vi "FP RT main.vi"() -> ()   [LabVIEW 2014]
uses:
  <vilib>/userdefined/High Color/IMAQdx.ctl
  <vilib>/myRIO/Instrument Drivers/Onboard IO/PWM/typedefs/PWM Reference.ctl
  <vilib>/myRIO/Common/Instrument Driver Framework/Utilities/typedefs/myRIO Generic Hardware Reference.ctl
  <vilib>/myRIO/Common/Instrument Driver Framework/Utilities/typedefs/Hardware Version Enum.ctl
  <vilib>/myRIO/Common/Instrument Driver Framework/Utilities/typedefs/myRIO v1.0 Reference.ctl
  <vilib>/myRIO/Common/Instrument Driver Framework/Utilities/typedefs/Generic FPGA Reference.ctl
  <vilib>/myRIO/Common/Instrument Driver Framework/myRIO v1.0/PWM/typedefs/PWM Channels Enum.ctl
  <vilib>/myRIO/Instrument Drivers/Onboard IO/PWM/typedefs/PWM Configuration.ctl
  <vilib>/userdefined/High Color/nirio_resource_hc.ctl
  <vilib>/myRIO/Instrument Drivers/Onboard IO/DIO/typedefs/DIO Reference.ctl
  <vilib>/myRIO/Common/Instrument Driver Framework/myRIO v1.0/DIO/typedefs/DIO Channels List.ctl
  <vilib>/myRIO/Common/Instrument Driver Framework/myRIO v1.0/DIO/typedefs/DIO Channels Enum.ctl
  <vilib>/myRIO/Instrument Drivers/Onboard IO/AI/typedefs/AI Reference.ctl
  <vilib>/myRIO/Common/Instrument Driver Framework/myRIO v1.0/AI/typedefs/AI Channels List.ctl
  <vilib>/myRIO/Common/Instrument Driver Framework/myRIO v1.0/AI/typedefs/AI Channels Enum.ctl
  <vilib>/myRIO/Common/Instrument Driver Framework/Utilities/typedefs/Analog Scaling Constants List.ctl
  <vilib>/myRIO/Common/Instrument Driver Framework/Utilities/typedefs/Analog Scaling Constants.ctl
  <vilib>/myRIO/Common/Instrument Driver Framework/myRIO v1.0/PWM/vis/myRIO v1.1 Open PWM.vi
  <vilib>/myRIO/Common/Instrument Driver Framework/myRIO v1.0/DIO/vis/myRIO v1.1 Open DIO.vi
  <vilib>/myRIO/Common/Instrument Driver Framework/myRIO v1.0/AI/vis/myRIO v1.1 Open AI.vi
  <vilib>/myRIO/Common/Instrument Driver Framework/Utilities/vis/Validate Channels.vi
  <vilib>/myRIO/Common/Instrument Driver Framework/myRIO v1.0/PWM/vis/myRIO v1.0 Reserve PWM.vi
  <vilib>/myRIO/Common/Instrument Driver Framework/myRIO v1.0/DIO/vis/myRIO v1.0 Reserve DIO.vi
  <vilib>/myRIO/Common/Instrument Driver Framework/myRIO v1.0/AI/vis/myRIO v1.0 Reserve AI.vi
  <vilib>/myRIO/Common/Instrument Driver Framework/myRIO v1.0/PWM/vis/myRIO v1.0 Close PWM.vi
  <vilib>/myRIO/Common/Instrument Driver Framework/myRIO v1.0/DIO/vis/myRIO v1.0 Close DIO.vi
  <vilib>/myRIO/Common/Instrument Driver Framework/myRIO v1.0/AI/vis/myRIO v1.0 Close AI.vi
  <vilib>/myRIO/Common/Instrument Driver Framework/myRIO v1.0/PWM/vis/myRIO v1.0 Build MUX Configuration PWM.vi
  <vilib>/myRIO/Common/Instrument Driver Framework/myRIO v1.0/Resource Manager/vis/myRIO v1.0 Reserve Channel List.vi
  <vilib>/myRIO/Common/Instrument Driver Framework/myRIO v1.0/DIO/vis/myRIO v1.0 Build MUX Configuration DIO.vi
  <vilib>/myRIO/Common/Instrument Driver Framework/myRIO v1.0/AI/vis/myRIO v1.0 Build MUX Configuration AI.vi
  <vilib>/myRIO/Common/Instrument Driver Framework/myRIO v1.0/PWM/vis/myRIO v1.0 Unreserve PWM.vi
  <vilib>/myRIO/Common/Instrument Driver Framework/myRIO v1.0/DIO/vis/myRIO v1.0 Unreserve DIO.vi
  <vilib>/myRIO/Common/Instrument Driver Framework/myRIO v1.0/AI/vis/myRIO v1.0 Unreserve AI.vi
  <vilib>/myRIO/Common/Instrument Driver Framework/myRIO v1.0/Resource Manager/vis/myRIO v1.0 Create Configuration List.vi
  <vilib>/myRIO/Common/Instrument Driver Framework/myRIO v1.0/Resource Manager/vis/myRIO v1.0 Reserve Channel.vi
  <vilib>/myRIO/Common/Instrument Driver Framework/myRIO v1.0/Resource Manager/vis/myRIO v1.0 Unreserve Channel.vi
  <vilib>/myRIO/Common/Instrument Driver Framework/myRIO v1.0/Resource Manager/vis/myRIO v1.0 Unreserve Channel List.vi
  <vilib>/myRIO/Common/Instrument Driver Framework/myRIO v1.0/Resource Manager/vis/myRIO v1.0 Build Mutex Name.vi
  <vilib>/Utility/VariantDataType/GetNumericInfo.vi
  <vilib>/Utility/error.llb/Error Cluster From Error Code.vi
  <vilib>/myRIO/Common/Instrument Driver Framework/myRIO v1.0/myRIO v1.1 Open.vi
  <vilib>/myRIO/Common/Instrument Driver Framework/myRIO v1.0/AI/vis/myRIO v1.0 Get Scaling Constants AI.vi
  <vilib>/myRIO/Common/Instrument Driver Framework/Utilities/vis/IO Manager.vi
  <vilib>/myRIO/Common/Instrument Driver Framework/Utilities/vis/Configuration Manager.vi
  <vilib>/myRIO/Common/Instrument Driver Framework/myRIO v1.0/myRIO v1.0 Close.vi
  <vilib>/myRIO/Common/Instrument Driver Framework/myRIO v1.0/Resource Manager/vis/myRIO v1.0 Configure IO.vi
  <vilib>/myRIO/Common/Instrument Driver Framework/myRIO v1.0/AI/vis/myRIO v1.0 Read AI.vi
  <vilib>/myRIO/Common/Instrument Driver Framework/myRIO v1.0/DIO/vis/myRIO v1.0 Write DIO.vi
  <vilib>/myRIO/Common/Instrument Driver Framework/myRIO v1.0/PWM/vis/myRIO v1.0 Write PWM.vi
  <vilib>/myRIO/Common/Instrument Driver Framework/myRIO v1.0/PWM/vis/myRIO v1.0 Shutdown PWM.vi
  <vilib>/myRIO/Common/Instrument Driver Framework/myRIO v1.0/DIO/vis/myRIO v1.0 Shutdown DIO.vi
  <vilib>/myRIO/Instrument Drivers/Onboard IO/AI/vis/myRIO AI Open.xnode
  <vilib>/myRIO/Instrument Drivers/Onboard IO/DIO/vis/myRIO DIO Open.xnode
  <vilib>/myRIO/Instrument Drivers/Onboard IO/PWM/vis/myRIO PWM Open.xnode
  <vilib>/vision/driver/NI_Vision_Acquisition_Software.lvlib
  <vilib>/myRIO/Instrument Drivers/Onboard IO/AI/AI.lvlib
  <vilib>/myRIO/Instrument Drivers/Onboard IO/DIO/DIO.lvlib
  <vilib>/myRIO/Instrument Drivers/Onboard IO/PWM/PWM.lvlib
panel:
  in  "Tab Control":T1(tab)
  out "GLED":bool
  out "BLED":bool
  out "RLED":bool
  out "BW Image":T2(plugin-control)
  in  "stop":bool
  out "Midbrain?":bool
  out "Rudder":dbl(knob) min=-45.0 max=45.0 step=1.0 scale=-45.0..45.0
  out "Speed":dbl(knob) min=-9.0 max=9.0 step=1.0 scale=-50.0..50.0
  out "Hindbrain?":bool
  out "Forebrain?":bool
  out "Battery Dead?":bool
  out "Complete?":bool=TRUE
  out "Arbiter Graph":cluster{dbl, dbl, dbl[]}(graph)
  in  "Session In":T3="cam0"
  out "Color Image":T2(plugin-control)
  out "Nb Circles":i32
  out "UDP Time Out?":bool
  in  "Tug letter":string="T"
  in  "Run?":bool
  in  "MSpeed":dbl(slide) scale=-50.0..50.0 scale format="%#.1g"
  in  "MHeading":dbl(slide) scale=-45.0..45.0 scale format="%_1f"
  in  "Manual?":bool
  out "Camera Data":T4(array[cluster])
  out "Boat Status":T5={"GPS"={"X pos"=0, "Y pos"=0, "Heading"=0.0}, "IR Sensors"=[{"Name"="Bow", "Angle"=0.0, "Distance"=0.0}], "MOT BAT"=7.2, "RIO BAT"=7.2}
  out "GPS?":bool
  out "Act Com":T6
  out "Forebrain ACT":dbl[](array[numeric])
  out "IR Sensors":T7(array[cluster])
  out "GPS":cluster{"X pos":i32, "Y pos":i32, "Heading":dbl}
  out "RED LED":bool
  out "GREEN LED":bool
  out "BLUE LED":bool
  in  "MDF":T8(array[cluster])=[{"Type"=enum."Start", "X"=250, "Y"=250, "Speed"=0, "Behaviors"=enum."Open Water Transit"}, {"Type"=enum."Waypoint", "X"=400, "Y"=100, "Speed"=20, "Behaviors"=enum."P-Wall Follow"}, {"Type"=enum."Waypoint", "X"=250, "Y"=250, "Speed"=20, "Behaviors"=enum."Open Water Transit"}, {"Type"=enum."Waypoint", "X"=250, "Y"=400, "Speed"=20, "Behaviors"=enum."Open Water Transit"}, {"Type"=enum."Waypoint", "X"=100, "Y"=400, "Speed"=20, "Behaviors"=enum."Open Water Transit"}, {"Type"=enum."End", "X"=250, "Y"=250, "Speed"=0, "Behaviors"=enum."Open Water Transit"}]
  out "GPS Initial":cluster{"X pos":i32, "Y pos":i32, "Heading":dbl}
  in  "Old Y Position":i32
  in  "Old X Position":i32
  out "Invalid Pos?":bool
  out "error out":errorcluster
  out "Forebrain Comd":T9
  out "Debug IR \nRaw \nReadings":T7(array[cluster])
  out "Boat Speed":dbl format="%#_15g"
  out "size(s)":i32
  out "MDF Active":T8(array[cluster])
  out "MDF INDEX":i32
  # "To start the Tug, press the \">\" key in the tool bar.\n\nPress the Run? control to start the Mission.\n\nWhen complete the Complete? indicator will light.\n\nIf the Run? is not pressed again, the mission will start again.\n\nAlways press the STOP button to end the operation!!!!!!!!!!!!!"
  # "Press the Manual? button to control\nthe Tug from the sliders"
  # "Stuck indicates that\nthe boat is not moving."
  # "Enter the Letter\nof  your Tug"
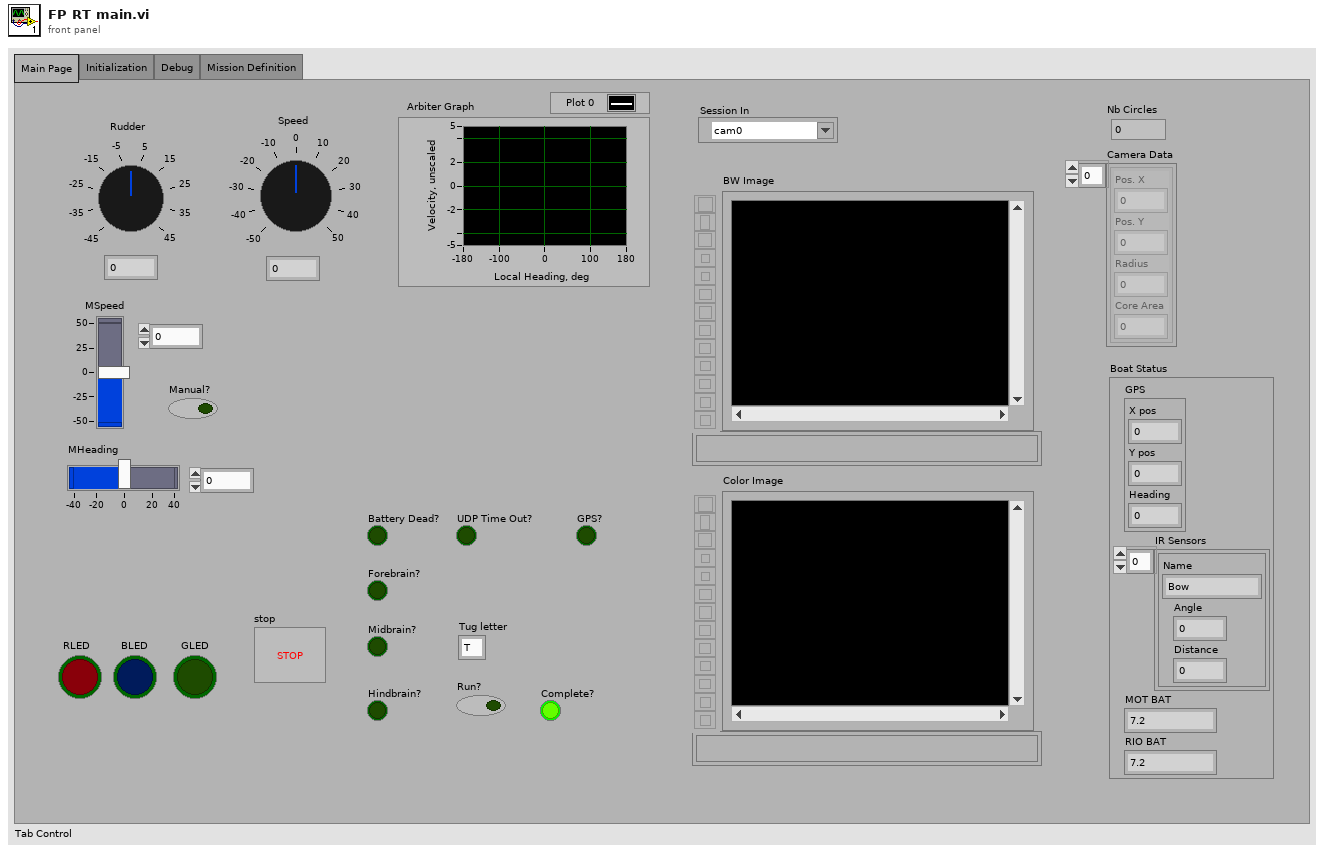
[diagram p1: front panel]
types:
  T1 = enum32{"Main Page", "Initialization", "Debug", "Mission Definition"}
  T2 = typedef "IMAQ Image.ctl" = refnum<image>
  T3 = typedef "IMAQdx.ctl" = refnum<k21>
  T4 = cluster{"Pos. X":i32, "Pos. Y":i32, "Radius":i32, "Core Area":i32}[]
  T5 = cluster{"GPS":cluster{"X pos":i32, "Y pos":i32, "Heading":dbl}, "IR Sensors":cluster{"Name":string, "Angle":dbl, "Distance":dbl}[], "MOT BAT":dbl, "RIO BAT":dbl}
  T6 = cluster{"Desired Local\nHeading":dbl, "Desired\nSpeed":dbl}
  T7 = cluster{"Name":string, "Angle":dbl, "Distance":dbl}[]
  T8 = cluster{"Type":enum16{"Start", "Waypoint", "End"}, "X":i32, "Y":i32, "Speed":i32, "Behaviors":enum16{"Open Water Transit", "P-Wall Follow", "S-Wall Follow", "Dock"}}[]
  T9 = cluster{"Behaviors":enum16{"Open Water Transit", "P-Wall Follow", "S-Wall Follow", "Dock"}, "Behavior\nVelocity":dbl}
  T10 = typedef "nirio_resource_hc.ctl" = tag
  T11 = typedef "Hardware Version Enum.ctl" = enum16{"Unknown", "myRIO-1900", "myRIO-1950"}
  T12 = typedef "Image Type" = u32
  T13 = enum16{"Open Water Transit", "P-Wall Follow", "S-Wall Follow", "Dock"}
  T14 = typedef "PWM.lvlib/PWM Reference.ctl" = cluster{"myRIO Reference":T15, "PWM Channels Enum":T18, "PWM Configuration":T19}
  T15 = typedef "myRIO Generic Hardware Reference.ctl" = cluster{"myRIO Model":T11, "myRIO Hardware Reference":T16}
  T16 = typedef "myRIO v1.0 Reference.ctl" = cluster{"Generic FPGA Reference":T17, "Allow multiple opens":bool}
  T17 = typedef "Generic FPGA Reference.ctl" = refnum<k20>
  T18 = typedef "PWM Channels Enum.ctl" = enum16{"Not Connected", "C/PWM0", "C/PWM1", "A/PWM0", "A/PWM1", "A/PWM2", "B/PWM0", "B/PWM1", "B/PWM2"}
  T19 = typedef "PWM.lvlib/PWM Configuration.ctl" = cluster{"Frequency":dbl, "Duty Cycle":dbl}
  T20 = typedef "DIO.lvlib/DIO Reference.ctl" = cluster{"myRIO Reference":T15, "DIO Channels List":T21}
  T21 = typedef "DIO Channels List.ctl" = T22[]
  T22 = typedef "DIO Channels Enum.ctl" = enum16{"Not Connected", "C/DIO0", "C/DIO1", "C/DIO2", "C/DIO3", "C/DIO4", "C/DIO5", "C/DIO6", "C/DIO7", "A/DIO0", "A/DIO1", "A/DIO2", "A/DIO3", "A/DIO4", "A/DIO5", "A/DIO6", "A/DIO7", "A/DIO8", "A/DIO9", "A/DIO10", "A/DIO11", "A/DIO12", "A/DIO13", "A/DIO14", "A/DIO15", "B/DIO0", "B/DIO1", "B/DIO2", "B/DIO3", "B/DIO4", "B/DIO5", "B/DIO6", "B/DIO7", "B/DIO8", "B/DIO9", "B/DIO10", "B/DIO11", "B/DIO12", "B/DIO13", "B/DIO14", "B/DIO15", "LED0", "LED1", "LED2", "LED3", "Button0"}
  T23 = typedef "AI.lvlib/AI Reference.ctl" = cluster{"myRIO Reference":T15, "AI Channels List":T24, "AI Scaling Constants List":T26}
  T24 = typedef "AI Channels List.ctl" = T25[]
  T25 = typedef "AI Channels Enum.ctl" = enum16{"Not Connected", "AudioIn/Left", "AudioIn/Right", "C/AI0", "C/AI1", "A/AI0", "A/AI1", "A/AI2", "A/AI3", "B/AI0", "B/AI1", "B/AI2", "B/AI3"}
  T26 = typedef "Analog Scaling Constants List.ctl" = T27[]
  T27 = typedef "Analog Scaling Constants.ctl" = cluster{"LSB Weight (Volts)":dbl, "Offset (Volts)":dbl, "Signed?":bool}
  T28 = cluster{"Obs Avoid Array":dbl[], "P-Wall Array":dbl[], "S-Wall Array":dbl[], "Unstuck Array":dbl[]}
  T29 = cluster{"regular expression":string, i32, i32, i32}
  T30 = cluster{"Behaviors":enum16{"Open Water Transit", "P-Wall Follow", "S-Wall Follow", "Dock"}, dbl}
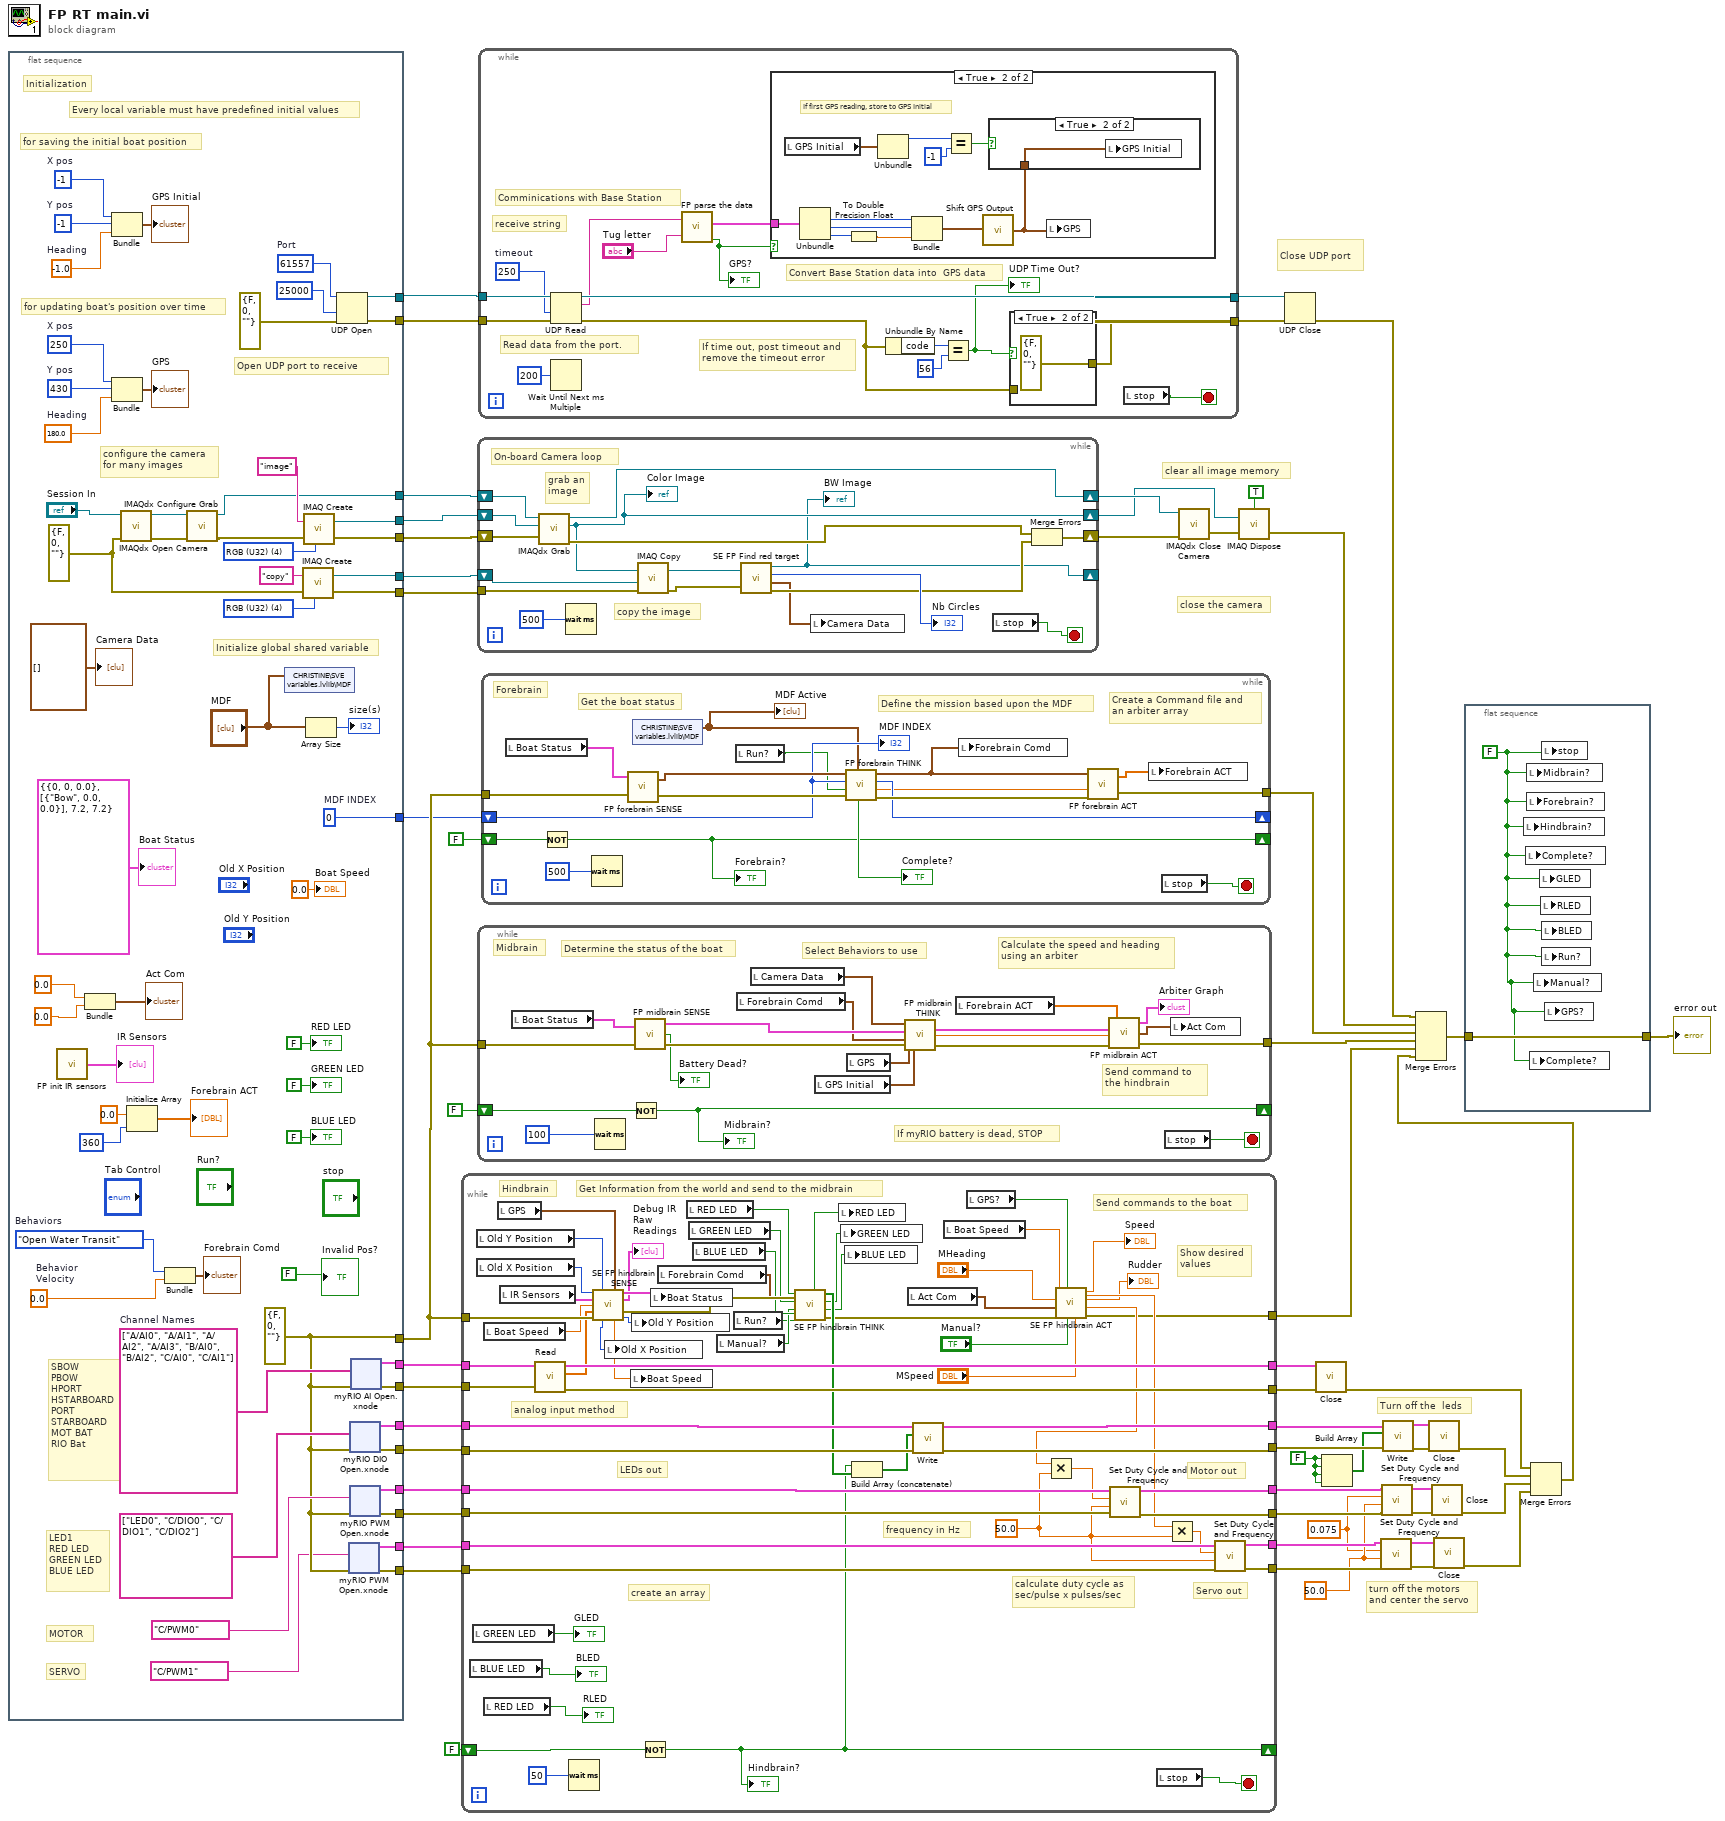
[diagram p0: block diagram]
diagram:
  w5 = 0.075
  w4 = FALSE
  w6 = 50.0
  # "Turn off the  leds"
  # "turn off the motors\nand center the servo"
  # "Close UDP port"
  # "clear all image memory"
  # "close the camera"
  n1 = flat-sequence {
    tunnel: [w74] -> w54
    tunnel: [w109] -> w51
    tunnel: [w100] -> w50
    tunnel: [w99] -> w49
    tunnel: [w98] -> w48
    tunnel: [w94] -> w41
    tunnel: [w93] -> w42
    tunnel: [w89] -> w36
    tunnel: [w88] -> w37
    tunnel: [w82] -> w34
    tunnel: [w81] -> w33
    tunnel: [w79] -> w29
    tunnel: [w78] -> w30
    tunnel: [w76] -> w28
    tunnel: [w75] -> w27
    tunnel: [w72] -> w26
    tunnel: [w71] -> w25
    frame #0 {
      w59 = -1  # Y pos
      w60 = -1  # X pos
      w61 = -1.0  # Heading
      w83 = tag[] ["A/AI0", "A/AI1", "A/AI2", "A/AI3", "B/AI0", "B/AI2", "C/AI0", "C/AI1"]  # Channel Names
      w85 = 430  # Y pos
      w86 = 250  # X pos
      w87 = 180.0  # Heading
      w92 = u16 61557  # Port
      w97 = T12 4 items=["Grayscale (U8)", "Grayscale (I16)", "Grayscale (SGL)", "Complex (CSG)", "RGB (U32)", "HSL (U32)", "RGB (U64)", "Grayscale (U16)"] ("Image Type")
      w95 = errorcluster {"status"=FALSE, "code"=0, "source"=""} ("error in")
      w105 = T12 4 items=["Grayscale (U8)", "Grayscale (I16)", "Grayscale (SGL)", "Complex (CSG)", "RGB (U32)", "HSL (U32)", "RGB (U64)", "Grayscale (U16)"] ("Image Type")
      w74 = errorcluster {"status"=FALSE, "code"=0, "source"=""} ("error out")
      w109 = 0  # MDF INDEX
      w113 = 0.0  # Behavior Velocity
      w108 = T13."Open Water Transit"  # Behaviors
      # "for saving the initial boat position"
      # "Initialize global shared variable"
      # "LED1\nRED LED\nGREEN LED\nBLUE LED"
      # "SERVO"
      # "MOTOR"
      # "SBOW\nPBOW\nHPORT\nHSTARBOARD\nPORT\nSTARBOARD\nMOT BAT\nRIO Bat"
      # "for updating boat's position over time"
      # "Open UDP port to receive"
      # "configure the camera\nfor many images"
      # "Every local variable must have predefined initial values"
      # "Initialization"
      n2 = call "FP init IR sensors.vi"() -> ("IR Sensors"=→"IR Sensors":T7)  [unwired: 1 in]
      n3 = Bundle(0.0, 0.0) -> (→"Act Com":cluster{dbl, dbl})  [unwired: 1 in]
      n4 = Bundle("X pos"=w60, "Y pos"=w59, "Heading"=w61) -> (→"GPS Initial":cluster{"X pos":i32, "Y pos":i32, "Heading":dbl})  [unwired: 1 in]
      n5 = Bundle("X pos"=w86, "Y pos"=w85, "Heading"=w87) -> (→"GPS":cluster{"X pos":i32, "Y pos":i32, "Heading":dbl})  [unwired: 1 in]
      n6 = call <vilib>:"IMAQdx Open Camera.vi"("error in"=w95, "Session In"="Session In") -> ("error out"=w102:errorcluster, "Session Out"=w101:T3)  [unwired: 1 in, 7 out]
      n7 = Initialize Array(0.0 ("element"), 360 ("dimension size")) -> (→"Forebrain ACT":dbl[])
      n8 = Bundle("Behaviors"=w108, "Behavior\nVelocity"=w113) -> (→"Forebrain Comd":T9)  [unwired: 1 in]
      n9 = call <vilib>:"IMAQdx Configure Grab.vi"("error in"=w102, "Session In"=w101) -> ("error out"=w106:errorcluster, "Session Out"=w98:T3)  [unwired: 8 out]
      n10 = shared-variable "CHRISTINE\\SVE variables.lvlib\\MDF"("MDF") -> ()  [unwired: 1 in, 1 out]
      n11 = call "IMAQ Create"("Image Name"="copy", "Image Type"=w97, "error in (no error)"=w95) -> ("New Image"=w93:T2, "error out"=w94:errorcluster)  [unwired: 2 in]
      n12 = call "IMAQ Create"("Image Name"="image", "Image Type"=w105, "error in (no error)"=w106) -> ("New Image"=w99:T2, "error out"=w100:errorcluster)  [unwired: 1 in, 1 out]
      n13 = Array Size(array="MDF") -> (size(s)=→"size(s)":i32)
      n14 = UDP Open(8:errorcluster {"status"=FALSE, "code"=0, "source"=""} ("error in"), 9:25000 ("timeout ms (25000)"), 11:w92) -> (port=w89:refnum<k16>, 0:w88:errorcluster)  [unwired: 2 in, 1 out]
      n15 = xnode "myRIO PWM Open.xnode"("error in (no error)"=w74, "Channel Name"=tag "C/PWM1") -> ("error out"=w72:errorcluster, "PWM Ref Out"=w71:T14)  [unwired: 1 in]
      n16 = xnode "myRIO DIO Open.xnode"("error in (no error)"=w74, "Channel Names"=tag[] ["LED0", "C/DIO0", "C/DIO1", "C/DIO2"]) -> ("error out"=w79:errorcluster, "DIO Ref Out"=w78:T20)  [unwired: 1 in]
      n17 = xnode "myRIO PWM Open.xnode"("error in (no error)"=w74, "Channel Name"=tag "C/PWM0") -> ("error out"=w76:errorcluster, "PWM Ref Out"=w75:T14)  [unwired: 1 in]
      n18 = xnode "myRIO AI Open.xnode"("error in (no error)"=w74, "Channel Names"=w83) -> ("error out"=w82:errorcluster, "AI Ref Out"=w81:T23)  [unwired: 1 in]
      "Invalid Pos?" <- FALSE
      "RED LED" <- FALSE ("RED LED")
      "GREEN LED" <- FALSE ("GREEN LED")
      "BLUE LED" <- FALSE ("WHITE LED")
      "Camera Data" <- T4 [] ("Camera Data")
      "Boat Status" <- T5 {"GPS"={"X pos"=0, "Y pos"=0, "Heading"=0.0}, "IR Sensors"=[{"Name"="Bow", "Angle"=0.0, "Distance"=0.0}], "MOT BAT"=7.2, "RIO BAT"=7.2} ("Boat Status 2")
      "Boat Speed" <- 0.0 ("Boat Speed")
    }
  }
  n19 = while {
    tunnel: w54 -> [w243]
    shift-right: [w207] -> _
    shift-left: FALSE -> [w232]
    tunnel: w34 -> [w240]
    tunnel: w33 -> [w239]
    tunnel: [w238] -> w32
    tunnel: [w237] -> w31
    tunnel: w30 -> [w235]
    tunnel: w29 -> [w236]
    tunnel: [w234] -> w11
    tunnel: [w233] -> w8
    tunnel: w28 -> [w230]
    tunnel: w27 -> [w231]
    tunnel: [w229] -> w20
    tunnel: [w228] -> w17
    tunnel: w26 -> [w227]
    tunnel: [w226] -> w24
    tunnel: w25 -> [w225]
    tunnel: [w224] -> w22
    tunnel: [w186] -> w1
    stop <- w245 stop-if-true
    w219 = 50.0
    # "create an array"
    # "frequency in Hz"
    # "calculate duty cycle as\nsec/pulse x pulses/sec"
    # "Show desired\nvalues"
    # "Motor out"
    # "Servo out"
    # "LEDs out"
    # "analog input method"
    # "Send commands to the boat"
    # "Get Information from the world and send to the midbrain"
    # "Hindbrain"
    n20 = local read "BLUE LED"() -> (→"BLED":bool)
    n21 = local read "GREEN LED"() -> (→"GLED":bool)
    n22 = local read "Old Y Position"() -> (w191:i32)
    n23 = local read "Old X Position"() -> (w192:i32)
    n24 = local read "Boat Speed"() -> (w188:dbl)
    n25 = local read "RED LED"() -> (→"RLED":bool)
    n26 = local read "GPS"() -> (w241:cluster{"X pos":i32, "Y pos":i32, "Heading":dbl})
    n27 = local read "IR Sensors"() -> (w205:T7)
    n28 = call <vilib>:"Read.vi"("error in (no error)"=w240, "AI Ref In"=w239) -> ("error out"=w238:errorcluster, "Values"=w223:dbl[], "AI Ref Out"=w237:T23)  [unwired: 7 in]
    n29 = Wait (ms)(milliseconds to wait=u32 50) -> ()  [unwired: 1 out]
    n30 = call "SE FP hindbrain SENSE.vi"("Old X Position"=w192, "Old Y Position"=w191, "GPS"=w241, "IR Sensors"=w205, "Old Speed of Boat\nin Pixels/Sec"=w188, "Analog Input Values"=w223, "error in"=w243) -> ("Boat Status"=w206:T5, "IR Sensors 2"=→"Debug IR \nRaw \nReadings":T7, "error out"=w242:errorcluster, "New X Position"=w190:i32, "New Speed of Boat\nin Pixels/Sec"=w194:dbl, "New Y Position"=w189:i32)  [unwired: 3 in]
    n31 = local write "Old X Position"(w190) -> ()
    n32 = local write "Boat Speed"(w194) -> ()
    n33 = local write "Old Y Position"(w189) -> ()
    n34 = Not(x=w232) -> (.not. x?=w207:bool)
    "Hindbrain?" <- w207
    n35 = local write "Boat Status"(w206) -> ()
    n36 = local read "Forebrain Comd"() -> (w204:T9)
    n37 = local read "RED LED"() -> (w210:bool)
    n38 = local read "GREEN LED"() -> (w209:bool)
    n39 = local read "BLUE LED"() -> (w208:bool)
    n40 = local read "Manual?"() -> (w200:bool)
    n41 = local read "Run?"() -> (w195:bool)
    n42 = call "SE FP hindbrain THINK.vi"("error in"=w242, "BLUE LED"=w208, "Forebrain Comd"=w204, "RUN?"=w195, "MANUAL"=w200, "GREEN LED"=w209, "RED LED"=w210) -> ("error out"=w187:errorcluster, "BLUE LED OUT"=w201:bool, "GREEN LED OUT"=w202:bool, "LED array"=w212:bool[], "RED LED OUT"=w203:bool)
    n43 = local write "RED LED"(w203) -> ()
    n44 = local write "GREEN LED"(w202) -> ()
    n45 = local write "BLUE LED"(w201) -> ()
    n46 = Build Array (concatenate)(w207, w212) -> (w211:bool[])
    n47 = local read "Act Com"() -> (w216:T6)
    n48 = call <vilib>:"Write.vi"("error in (no error)"=w236, "Values"=w211, "DIO Ref In"=w235) -> ("error out"=w234:errorcluster, "DIO Ref Out"=w233:T20)  [unwired: 6 in]
    n49 = local read "Boat Speed"() -> (w193:dbl)
    n50 = local read "GPS?"() -> (w185:bool)
    n51 = call "SE FP hindbrain ACT.vi"("MSpeed"="MSpeed", "Manual?"="Manual?", "GPS?"=w185, "error in"=w187, "Act Com"=w216, "MHeading"="MHeading", "Current Boat Speed"=w193) -> ("error out"=w186:errorcluster, "Speed"=w222:dbl, "Desired \nRudder"=→"Rudder":dbl, "Desired\nSpeed"=→"Speed":dbl, "Rudder"=w220:dbl)
    n52 = Multiply(x=w222, y=w219) -> (x*y=w221:dbl)
    n53 = call <vilib>:"Set Duty Cycle and Frequency.vi"("error in (no error)"=w230, "Frequency [Hz]"=w219, "Duty Cycle"=w221, "PWM Ref In"=w231) -> ("error out"=w229:errorcluster, "PWM Ref Out"=w228:T14)  [unwired: 5 in]
    n54 = local read "stop"() -> (w245:bool)
    n55 = Multiply(x=w220, y=w219) -> (x*y=w218:dbl)
    n56 = call <vilib>:"Set Duty Cycle and Frequency.vi"("error in (no error)"=w227, "Frequency [Hz]"=w219, "Duty Cycle"=w218, "PWM Ref In"=w225) -> ("error out"=w226:errorcluster, "PWM Ref Out"=w224:T14)  [unwired: 5 in]
  }
  n57 = while {
    shift-right: [w249] -> w46
    shift-left: w50 -> [w261]
    shift-right: [w248] -> w44
    shift-left: w49 -> [w260]
    shift-right: [w253] -> w45
    shift-left: w48 -> [w259]
    tunnel: w41 -> [w257]
    shift-right: [w247] -> _
    shift-left: w42 -> [w256]
    stop <- w262 stop-if-true
    # "grab an\nimage"
    # "copy the image"
    # "On-board Camera loop"
    n58 = call <vilib>:"IMAQdx Grab.vi"("error in"=w261, "Image In"=w260, "Session In"=w259) -> ("error out"=w250:errorcluster, "Image Out"=w248:T2, "Session Out"=w253:T3)  [unwired: 5 in, 1 out]
    "Color Image" <- w248
    n59 = Wait (ms)(milliseconds to wait=u32 500) -> ()  [unwired: 1 out]
    n60 = call "IMAQ Copy"("error in (no error)"=w257, "Image Dst"=w256, "Image Src"=w248) -> ("error out"=w255:errorcluster, "Image Dst Out"=w254:T2)  [unwired: 3 in]
    n61 = call "SE FP Find red target.vi"("Image In"=w254, "error in (no error)"=w255) -> ("Image Dst Out"=w247:T2, "Nb Circles (Circle Detection 1)"=→"Nb Circles":i32, "Camera Data"=w246:T4, "error out"=w251:errorcluster)
    "BW Image" <- w247
    n62 = local write "Camera Data"(w246) -> ()
    n63 = local read "stop"() -> (w262:bool)
    n64 = Merge Errors(w250, w251) -> (w249:errorcluster)
  }
  n65 = while {
    shift-right: [w270] -> _
    shift-left: FALSE -> [w281]
    tunnel: w54 -> [w280]
    tunnel: [w274] -> w56
    stop <- w282 stop-if-true
    # "If myRIO battery is dead, STOP"
    # "Send command to \nthe hindbrain"
    # "Calculate the speed and heading\nusing an arbiter"
    # "Select Behaviors to use"
    # "Determine the status of the boat"
    # "Midbrain"
    n66 = local read "Boat Status"() -> (w265:T5)
    n67 = Wait (ms)(milliseconds to wait=u32 100) -> ()  [unwired: 1 out]
    n68 = Not(x=w281) -> (.not. x?=w270:bool)
    "Midbrain?" <- w270
    n69 = call "FP midbrain SENSE.vi"("Boat Status"=w265, "error in"=w280) -> ("IR Sensors"=w268:T7, "Battery\nDead?"=→"Battery Dead?":bool, "error out"=w278:errorcluster)
    n70 = local read "Forebrain Comd"() -> (w267:T9)
    n71 = local read "Camera Data"() -> (w266:T4)
    n72 = local read "GPS Initial"() -> (w264:cluster{"X pos":i32, "Y pos":i32, "Heading":dbl})
    n73 = local read "GPS"() -> (w263:cluster{"X pos":i32, "Y pos":i32, "Heading":dbl})
    n74 = call "FP midbrain THINK.vi"("Camera Data"=w266, "error in"=w278, "IR Sensors"=w268, "Forebrain Comd"=w267, "GPS  Initial"=w264, "GPS"=w263) -> ("Behavior arrays"=w275:T28, "Behavior\nVelocity OUT"=w272:dbl, "error out"=w277:errorcluster)
    n75 = local read "Forebrain ACT"() -> (w273:dbl[])
    n76 = call "FP midbrain ACT.vi"("error in"=w277, "Behavior\nVelocity"=w272, "Behavior arrays"=w275, "Forebrain ACT"=w273) -> ("error out"=w274:errorcluster, "Act Com"=w279:T6, "Waveform Graph"=→"Arbiter Graph":cluster{dbl, dbl, dbl[]})
    n77 = local read "stop"() -> (w282:bool)
    n78 = local write "Act Com"(w279) -> ()
  }
  n79 = while {
    tunnel: w37 -> [w297]
    tunnel: w36 -> [w296]
    tunnel: [w295] -> w39
    tunnel: [w290] -> w38
    stop <- w287 stop-if-true
    w289 = 250  # timeout
    # "Convert Base Station data into  GPS data"
    # "Comminications with Base Station"
    # "receive string"
    # "If time out, post timeout and\nremove the timeout error"
    # "Read data from the port."
    n80 = UDP Read(connection ID=w296, timeout ms (25000)=w289, 8:w297) -> (data out=w284:string, error out=w291:errorcluster, 3:w295:refnum<k16>)  [unwired: 1 in, 2 out]
    n81 = Wait Until Next ms Multiple(millisecond multiple=u32 200) -> ()  [unwired: 1 out]
    n82 = call "FP parse the data.vi"("Nav String"=w284, "Tug"="Tug letter") -> ("Tug Location"=w285:T29, "Valid?"=w283:bool)  [unwired: 2 out]
    "GPS?" <- w283
    n83 = case shown="True" w283 {
      tunnel: w285 -> [_ w308]
      frame False {
      }
      frame True {
        # "If first GPS reading, store to GPS Initial"
        n84 = local read "GPS Initial"() -> (w301:cluster{"X pos":i32, "Y pos":i32, "Heading":dbl})
        n85 = Unbundle(w308) -> (w307:i32, w306:i32, w304:i32)  [unwired: 1 out]
        n86 = To Double Precision Float(number=w304) -> (double precision float=w305:dbl)
        n87 = Unbundle(w301) -> ("X pos"=w300:i32)  [unwired: 2 out]
        n88 = Bundle(w307, w306, w305) -> (w303:cluster{i32, i32, dbl})  [unwired: 1 in]
        n89 = Equal?(x=w300, y=-1) -> (x = y?=w299:bool)
        n90 = call "Shift GPS Output.vi"("GPS Input"=w303) -> ("GPS Output"=w302:cluster{"X pos":i32, "Y pos":i32, "Heading":dbl})
        n91 = case shown="True" w299 {
          tunnel: w302 -> [_ w309]
          frame False {
          }
          frame True {
            n92 = local write "GPS Initial"(w309) -> ()
          }
        }
        n93 = local write "GPS"(w302) -> ()
      }
    }
    n94 = Unbundle By Name(w291) -> ("code"=w294:i32)
    n95 = Equal?(x=w294, y=56) -> (x = y?=w292:bool)
    "UDP Time Out?" <- w292
    n96 = case shown="True" w292 {
      tunnel: [w310 errorcluster {"status"=FALSE, "code"=0, "source"=""} ("error out")] -> w290
      tunnel: w291 -> [w310 _]
      frame False {
      }
      frame True {
      }
    }
    n97 = local read "stop"() -> (w287:bool)
  }
  n98 = while {
    tunnel: w54 -> [w327]
    shift-right: [w315] -> _
    shift-left: FALSE -> [w316]
    tunnel: [w324] -> w52
    shift-right: [w320] -> _
    shift-left: w51 -> [w318]
    stop <- w328 stop-if-true
    # "Create a Command file and \nan arbiter array"
    # "Define the mission based upon the MDF"
    # "Get the boat status"
    # "Forebrain"
    n99 = local read "Boat Status"() -> (w322:T5)
    n100 = Not(x=w316) -> (.not. x?=w315:bool)
    "Forebrain?" <- w315
    n101 = Wait (ms)(milliseconds to wait=u32 500) -> ()  [unwired: 1 out]
    n102 = call "FP forebrain SENSE.vi"("error in"=w327, "Boat Status"=w322) -> ("error out"=w326:errorcluster, "GPS"=w321:cluster{"X pos":i32, "Y pos":i32, "Heading":dbl})  [unwired: 1 in]
    n103 = shared-variable "CHRISTINE\\SVE variables.lvlib\\MDF"() -> (w312:T8)  [unwired: 1 in, 1 out]
    "MDF Active" <- w312
    n104 = local read "Run?"() -> (w314:bool)
    n105 = call "FP forebrain THINK.vi"("MDF in"=w312, "error in"=w326, "Run?"=w314, "MDF index"=w318, "GPS"=w321) -> ("error out"=w325:errorcluster, "local Steering\nangle"=w319:dbl, "MDF Index out"=w320:i32, "Behaviors out"=w313:T30, "Complete?"=→"Complete?":bool)
    n106 = local write "Forebrain Comd"(w313) -> ()
    n107 = call "FP forebrain ACT.vi"("error in"=w325, "local Steering\nangle"=w319, "Behaviors in"=w313) -> ("error out"=w324:errorcluster, "Forebrain ACT"=w323:dbl[])
    n108 = local write "Forebrain ACT"(w323) -> ()
    n109 = local read "stop"() -> (w328:bool)
    "MDF INDEX" <- w318
  }
  n110 = call <vilib>:"IMAQdx Close Camera.vi"("error in"=w46, "Session In"=w45) -> ("error out"=w47:errorcluster)  [unwired: 9 out]
  n111 = call "IMAQ Dispose"("All Images? (No)"=TRUE, "Image"=w44, "error in (no error)"=w47) -> ("error out"=w43:errorcluster)  [unwired: 3 out]
  n112 = UDP Close(connection ID=w39, 8:w38) -> (error out=w35:errorcluster)  [unwired: 1 out]
  n113 = call <vilib>:"Close.vi"("error in (no error)"=w32, "AI Ref In"=w31) -> ("error out"=w13:errorcluster)  [unwired: 9 in]
  n114 = Build Array(w4, w4, w4, w4) -> (w7:bool[])
  n115 = call <vilib>:"Set Duty Cycle and Frequency.vi"("error in (no error)"=w24, "Frequency [Hz]"=w6, "Duty Cycle"=w5, "PWM Ref In"=w22) -> ("error out"=w23:errorcluster, "PWM Ref Out"=w21:T14)  [unwired: 5 in]
  n116 = call <vilib>:"Set Duty Cycle and Frequency.vi"("error in (no error)"=w20, "Frequency [Hz]"=w6, "Duty Cycle"=w5, "PWM Ref In"=w17) -> ("error out"=w19:errorcluster, "PWM Ref Out"=w18:T14)  [unwired: 5 in]
  n117 = call <vilib>:"Write.vi"("error in (no error)"=w11, "Values"=w7, "DIO Ref In"=w8) -> ("error out"=w10:errorcluster, "DIO Ref Out"=w9:T20)  [unwired: 6 in]
  n118 = call <vilib>:"Close.vi"("error in (no error)"=w10, "DIO Ref In"=w9) -> ("error out"=w14:errorcluster)  [unwired: 9 in]
  n119 = call <vilib>:"Close.vi"("error in (no error)"=w19, "PWM Ref In"=w18) -> ("error out"=w15:errorcluster)  [unwired: 9 in]
  n120 = call <vilib>:"Close.vi"("error in (no error)"=w23, "PWM Ref In"=w21) -> ("error out"=w16:errorcluster)  [unwired: 9 in]
  n121 = flat-sequence {
    tunnel: [w331] -> w3
    tunnel: w2 -> [w331]
    frame #0 {
      w330 = FALSE
      n122 = local write "Hindbrain?"(w330) -> ()
      n123 = local write "Complete?"(w330) -> ()
      n124 = local write "Midbrain?"(w330) -> ()
      n125 = local write "Forebrain?"(w330) -> ()
      n126 = local write "Complete?"(w330) -> ()
      n127 = local write "Manual?"(w330) -> ()
      n128 = local write "GLED"(w330) -> ()
      n129 = local write "RLED"(w330) -> ()
      n130 = local write "stop"(w330) -> ()
      n131 = local write "BLED"(w330) -> ()
      n132 = local write "Run?"(w330) -> ()
      n133 = local write "GPS?"(w330) -> ()
    }
  }
  n134 = Merge Errors(w13, w14, w15, w16) -> (w12:errorcluster)
  n135 = Merge Errors(w35, w43, w52, w56, w1, w12) -> (w2:errorcluster)
  "error out" <- w3
